vi "change.vi"(1 "start":bool, 2 "back":bool) -> (0 "output":dbl)   [LabVIEW 2020]
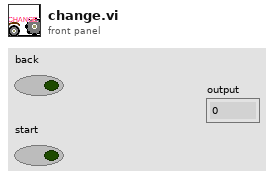
[diagram p1: front panel]
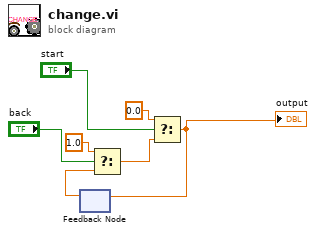
[diagram p0: block diagram]
diagram:
  n1 = feedback #1() -> (w6:dbl)  [unwired: 1 in]
  n2 = Select(t=1.0, s="back", f=w6) -> (s? t:f=w1:dbl)
  n3 = Select(t=0.0, s="start", f=w1) -> (s? t:f=w3:dbl)
  "output" <- w3
  n4 = feedback-in #1(w3) -> ()
